vi "Protocol.Initialize.vi"(8 "error in (no error)":errorcluster, 10 "Parameters in":T8={"Name"="", "XNET.Settings"={"Database"="", "Cluster"="", "Port"="", "Baud rate [Bd]"=0, "Termination"=0, "Incoming Decimation"=0, "Outgoing Decimation"=1}, "Monitor.Network"={"Address"=0, "Name"=0, "Include DA"=FALSE}, "Data"=[], "DTCs"=[], "Sim.Nodes.LUT"=variant, "Data.LUT"=variant} {"Monitor.Network"."Name" format="%.0x"; "DTCs"."Data"."DM1.Ref"."Data Reference" format="%.0x"; "DTCs"."Data"."DM1.Enable.Ref"."Data Reference" format="%.0x"; "DTCs"."Data"."DM2.Ref"."Data Reference" format="%.0x"; "DTCs"."Data"."DM2.Enable.Ref"."Data Reference" format="%.0x"; "Data"."Trigger.Refs"."Data Reference" format="%.0x"; "Data"."Disable.Refs"."Data Reference" format="%.0x"; "Data"."Timing.Refs"."Data Reference" format="%.0x"; "Data"."Network"."Name" format="%.0x"; "Data"."Incoming.Refs"."Data Reference" format="%.0x"; "Data"."Outgoing.Refs"."Data Reference" format="%.0x"; "XNET.Settings"."Termination" items=["Off", "On"]}, 11 "Process":refnum<class "Process.lvclass">) -> (0 "error out":errorcluster, 2 "Notification":bool, 3 "J1939 Main Configuration":T1)   [LabVIEW 2015, in "J1939 Addon Engine.lvlib"]
uses:
  J1939 Addon Engine.lvlib
  Types/Protocol.App Settings.ctl
  Shared/Types/XNET Settings.ctl
  Shared/Types/Monitor Settings.ctl
  Types/Protocol.XNET Refs.ctl
  <vilib>/NI Veristand/Custom Device API/Block Data Reference.ctl
  <vilib>/NI Veristand/Custom Device API/Data Reference.ctl
  Types/Main.Outgoing.Frame.Settings.ctl
  Shared/Types/Outgoing Event Trigger Types.ctl
  Types/Engine.DTC Settings.ctl
  Shared/Types/Compiled Simulated Settings.ctl
  Types/Engine.DTC FIFOs.ctl
  Types/Protocol.Configuration.ctl
  <vilib>/NI/NIVS Inline Async API/_VS Inline Async API/Process/Process.lvclass
  <vilib>/NI/NIVS Addon Network Comm/Engine/VeriStand Comm.lvclass
  Types/Protocol.Refs.ctl
  Shared/J1939 Utilities/Types/CAN Outgoing Message Cluster.ctl
  Types/Protocol.RQST Lookup Table Reference.ctl
  Types/Protocol.Address Table Reference.ctl
  Types/Protocol.XNET Settings.ctl
  <vilib>/NI/NIVS Inline Async API/_Data Access Engine/Data Access Engine/Types/Read.DVR.ctl
  <vilib>/NI/NIVS Inline Async API/_Data Access Engine/Access Type Classes/Read/Read.lvclass
  <vilib>/NI/NIVS Inline Async API/_Data Access Engine/Data Access Engine/Types/Write.DVR.ctl
  <vilib>/NI/NIVS Inline Async API/_Data Access Engine/Access Type Classes/Write/Write.lvclass
  <vilib>/NI/NIVS Addon Network Comm/Engine/VeriStand Comm.lvclass/VeriStand Comm.ctl
  <vilib>/NI/NIVS Inline Async API/_VS Inline Async API/Process/Process.lvclass/Process.ctl
  <vilib>/NI/NIVS Inline Async API/_VS Inline Async API/Process/Data Member Access/Read Data Access.vi
  <vilib>/NI/NIVS Inline Async API/_VS Inline Async API/Error Handling Process/SubVIs/Error.ConvertArray.vi
  <vilib>/NI/NIVS Inline Async API/_Data Access Engine/Data Access Engine/Methods/Write.Lookup.vi
  <vilib>/NI/NIVS Inline Async API/_Data Access Engine/Data Access Engine/Methods/Read.Lookup.vi
  <vilib>/NI/STM/Connection Manager/TCP/Advanced/TCP Initialize Connection Manager (By Reference).vi
  <vilib>/NI/AMC/Create Message Queue.vi
  Shared/SubVIs/Constants.vi
  <vilib>/NI/NIVS Inline Async API/_Data Access Engine/Data Access Engine/Data Access Engine.lvclass
  Shared/J1939 Utilities/J1939 Utilities.lvlib
  <vilib>/NI VeriStand/Custom Device Tools/Custom Device Utility Library/Custom Device Utility Library.lvlib
  Shared/J1939 Addon Shared.lvlib
  <vilib>/NI VeriStand/Custom Device API/Custom Device API.lvlib
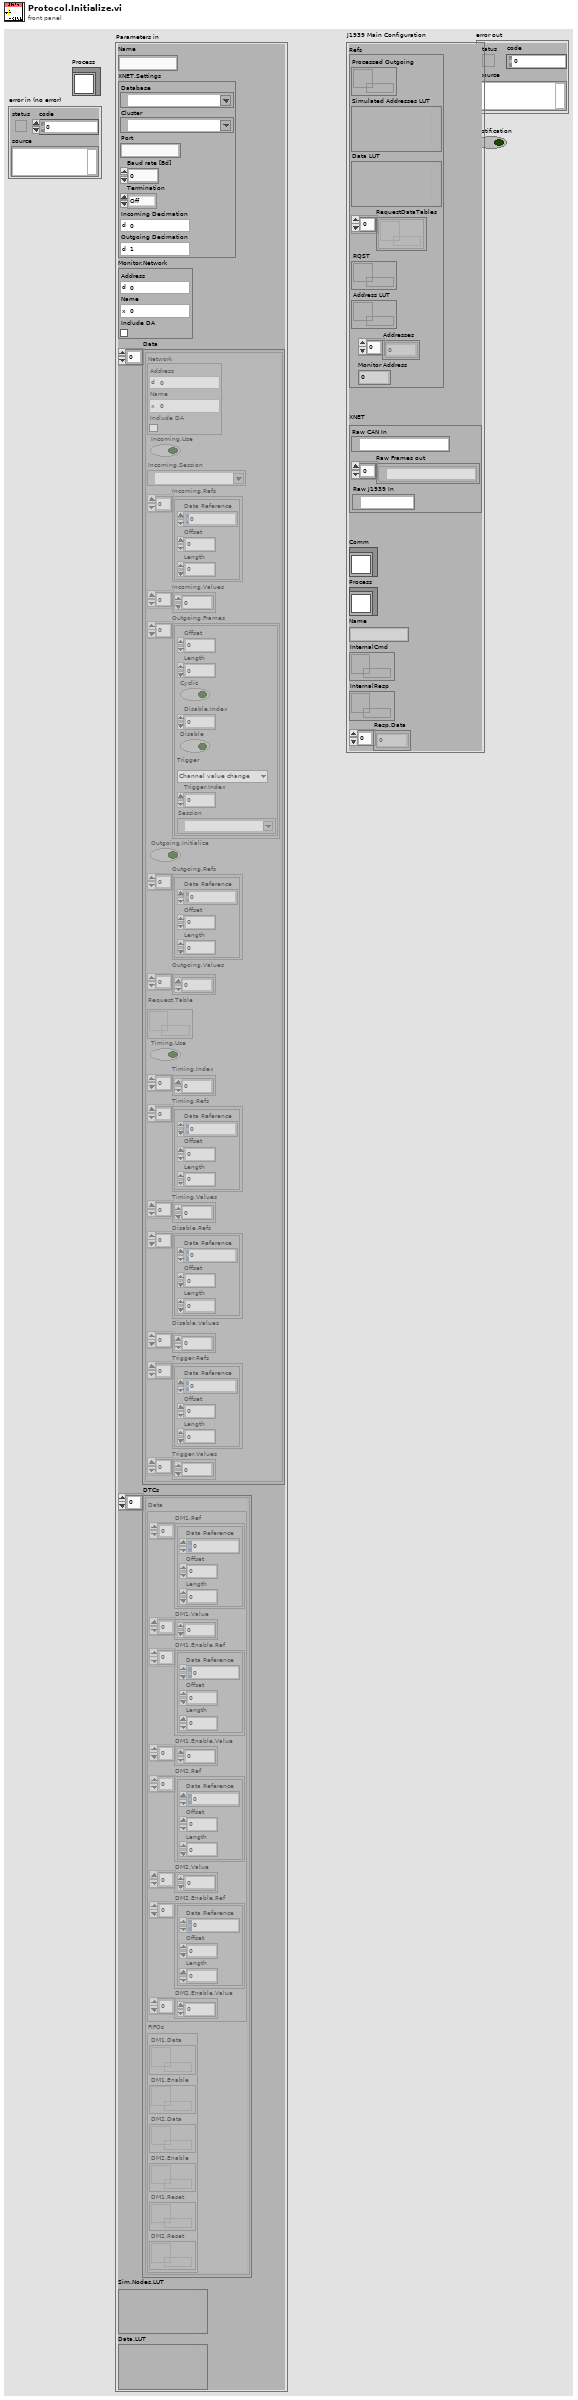
[diagram p1: front panel]
types:
  T1 = typedef "J1939 Addon Engine.lvlib/Protocol.Configuration.ctl" = cluster{"Refs":T2, "XNET":T5, "Comm":refnum<class "VeriStand Comm.lvclass">, "Process":refnum<class "Process.lvclass">, "Name":string, "InternalCmd":T6, "InternalResp":T7, "Resp.Data":dbl[]}
  T2 = typedef "J1939 Addon Engine.lvlib/Protocol.Refs.ctl" = cluster{"Processed Outgoing":refnum<queue>, "Simulated Addresses LUT":variant, "Data LUT":variant, "RequestDataTables":refnum<k33>[], "RQST":T3, "Address LUT":T4, "Addresses":u8[], "Monitor Address":u8}
  T3 = typedef "J1939 Addon Engine.lvlib/Protocol.RQST Lookup Table Reference.ctl" = refnum<data-value>
  T4 = typedef "J1939 Addon Engine.lvlib/Protocol.Address Table Reference.ctl" = refnum<data-value>
  T5 = typedef "J1939 Addon Engine.lvlib/Protocol.XNET Settings.ctl" = cluster{"Raw CAN In":refnum<k21>, "Raw Frames out":refnum<k21>[], "Raw J1939 In":refnum<k21>}
  T6 = typedef "Data Access Engine.lvlib/Data Access Engine.lvclass/Read.DVR.ctl" = refnum<data-value>
  T7 = typedef "Data Access Engine.lvlib/Data Access Engine.lvclass/Write.DVR.ctl" = refnum<data-value>
  T8 = typedef "J1939 Addon Engine.lvlib/Protocol.App Settings.ctl" = cluster{"Name":string, "XNET.Settings":T9, "Monitor.Network":T10, "Data":T11[], "DTCs":T16[], "Sim.Nodes.LUT":variant, "Data.LUT":variant}
  T9 = typedef "J1939 Addon Shared.lvlib/XNET Settings.ctl" = cluster{"Database":refnum<k21>, "Cluster":refnum<k21>, "Port":string, "Baud rate [Bd]":u32, "Termination":u32, "Incoming Decimation":u32, "Outgoing Decimation":u32}
  T10 = typedef "J1939 Addon Shared.lvlib/Monitor Settings.ctl" = cluster{"Address":u8, "Name":u64, "Include DA":bool}
  T11 = typedef "J1939 Addon Engine.lvlib/Protocol.XNET Refs.ctl" = cluster{"Network":T10, "Incoming.Use":bool, "Incoming.Session":refnum<k21>, "Incoming.Refs":T12[], "Incoming.Values":dbl[], "Outgoing.Frames":T14[], "Outgoing.Initialize":bool, "Outgoing.Refs":T12[], "Outgoing.Values":dbl[], "Request.Table":refnum<k33>, "Timing.Use":bool, "Timing.Index":i32[], "Timing.Refs":T12[], "Timing.Values":dbl[], "Disable.Refs":T12[], "Disable.Values":dbl[], "Trigger.Refs":T12[], "Trigger.Values":dbl[]}
  T12 = typedef "Custom Device API.lvlib/Block Data Reference.ctl" = cluster{"Data Reference":T13, "Offset":u64, "Length":u64}
  T13 = typedef "Custom Device API.lvlib/Data Reference.ctl" = i32
  T14 = typedef "J1939 Addon Engine.lvlib/Main.Outgoing.Frame.Settings.ctl" = cluster{"Offset":u32, "Length":u32, "Cyclic":bool, "Disable.Index":i32, "Disable":bool, "Trigger":T15, "Trigger.Index":i32, "Session":refnum<k21>}
  T15 = typedef "J1939 Addon Shared.lvlib/Outgoing Event Trigger Types.ctl" = enum16{"Channel value change", "Trigger channel (not zero)", "Channel value change or trigger channel (not zero)", "Trigger channel (any value change)", "Channel value change or trigger channel (any value change)"}
  T16 = typedef "J1939 Addon Engine.lvlib/Engine.DTC Settings.ctl" = cluster{"Data":T17, "FIFOs":T18}
  T17 = typedef "J1939 Addon Shared.lvlib/Compiled Simulated Settings.ctl" = cluster{"DM1.Ref":T12[], "DM1.Value":dbl[], "DM1.Enable.Ref":T12[], "DM1.Enable.Value":dbl[], "DM2.Ref":T12[], "DM2.Value":dbl[], "DM2.Enable.Ref":T12[], "DM2.Enable.Value":dbl[]}
  T18 = typedef "J1939 Addon Engine.lvlib/Engine.DTC FIFOs.ctl" = cluster{"DM1.Data":refnum<k33>, "DM1.Enable":refnum<k33>, "DM2.Data":refnum<k33>, "DM2.Enable":refnum<k33>, "DM1.Reset":refnum<k33>, "DM2.Reset":refnum<k33>}
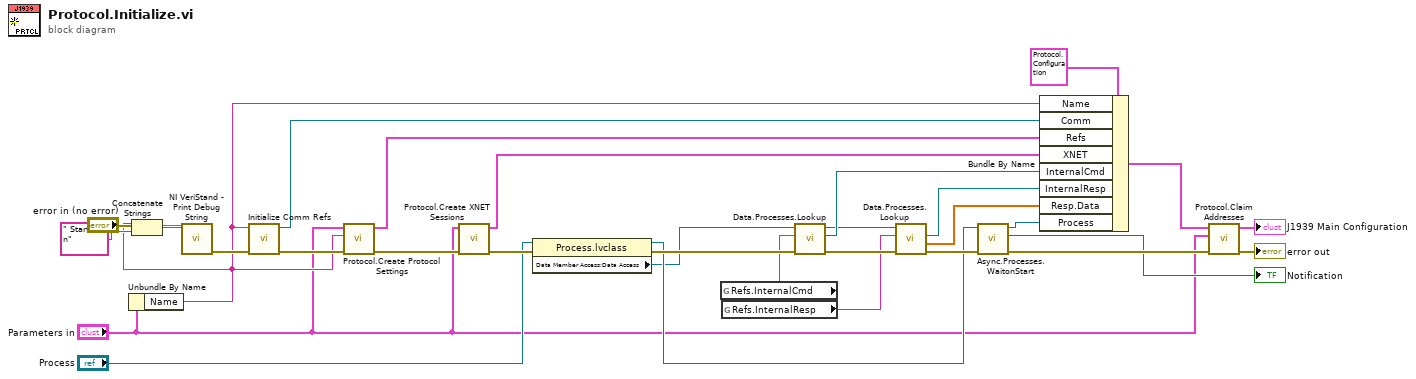
[diagram p0: block diagram]
diagram:
  n1 = Unbundle By Name("Parameters in") -> ("Name"=w3:string)
  n2 = Concatenate Strings(w3, " Started\n" ("string")) -> (w29:string)
  n3 = call <vilib>:"NI VeriStand - Print Debug String.vi"("error in (no error)"="error in (no error)", "Message"=w29) -> ("error out"=w24:errorcluster)  [unwired: 9 in]
  n4 = call <vilib>:"Initialize Comm Refs.vi"("error in (no error)"=w24, "Name"=w3) -> ("error out"=w23:errorcluster, "Comm.lvclass"=w22:refnum<class "VeriStand Comm.lvclass">)  [unwired: 8 in]
  n5 = call "Protocol.Create Protocol Settings.vi"("error in (no error)"=w23, "Name in"=w3, "Parameters in"="Parameters in") -> ("error out"=w28:errorcluster, "Protocol Refs"=w27:T2)  [unwired: 7 in]
  n6 = call "Protocol.Create XNET Sessions.vi"("error in (no error)"=w28, "Parameters in"="Parameters in") -> ("error out"=w10:errorcluster, "XNET"=w26:T5)  [unwired: 8 in]
  n7 = property class="Process.lvclass"(reference="Process", error in=w10) -> (reference out=w7:refnum<class "Process.lvclass">, error out=w9:errorcluster, "Data Member Access:Data Access"=w6:refnum<class "Data Access Engine.lvclass">)
  n8 = global read "Constants.vi" "Refs.InternalCmd"() -> (w4:string)
  n9 = global read "Constants.vi" "Refs.InternalResp"() -> (w5:string)
  n10 = call-poly <vilib>:"Data.Processes.Lookup.vi"("error in (no error)"=w9, "Name"=w4, "Data Access API in"=w6) -> ("error out"=w12:errorcluster, "Ref"=w15:T6, "Data Access API out"=w11:refnum<class "Data Access Engine.lvclass">)  [unwired: 5 in, 1 out]
  n11 = call-poly <vilib>:"Data.Processes.Lookup.vi"("error in (no error)"=w12, "Name"=w5, "Data Access API in"=w11) -> ("error out"=w13:errorcluster, "Initial Values"=w14:dbl[], "Ref"=w16:T7)  [unwired: 5 in, 1 out]
  n12 = call <vilib>:"Async.Processes.WaitonStart.vi"("error in (no error)"=w13, "Process"=w7) -> ("error out"=w21:errorcluster, "Execute"=→"Notification":bool, "Process out"=w19:refnum<class "Process.lvclass">)  [unwired: 7 in]
  n13 = Bundle By Name(cluster=T1 {"Refs"={"Processed Outgoing"=refnum, "Simulated Addresses LUT"=variant, "Data LUT"=variant, "RequestDataTables"=[], "RQST"=refnum, "Address LUT"=refnum, "Addresses"=[], "Monitor Address"=0}, "XNET"={"Raw CAN In"="", "Raw Frames out"=[], "Raw J1939 In"=""}, "Comm"=refnum, "Process"=refnum, "Name"="", "InternalCmd"=refnum, "InternalResp"=refnum, "Resp.Data"=[]} ("output cluster"), "Name"=w3, "Comm"=w22, "Refs"=w27, "XNET"=w26, "InternalCmd"=w15, "InternalResp"=w16, "Resp.Data"=w14, "Process"=w19) -> (w1:T1)
  n14 = call "Protocol.Claim Addresses.vi"("error in"=w21, "Parameters in"="Parameters in", "J1939 Main Configuration"=w1) -> ("error out"=→"error out":errorcluster, "output cluster"=→"J1939 Main Configuration":T1)  [unwired: 7 in]
